vi "TestObserveString_ValueHi.vi"(8 "error in (no error)":errorcluster, 11 "TestCase in":refnum<class "TestObservableData.lvclass">) -> (0 "error out":errorcluster, 3 "TestCase out":refnum<class "TestObservableData.lvclass">)   [LabVIEW 2015, in "TestObservableData.lvclass"]
uses:
  TestObservableData.lvclass
  TestObservableData.lvclass/TestObservableData.ctl
  Framework/IMediator/IMediator Messages/Subscribe Msg/Subscribe Msg.lvclass/Subscribe Msg.ctl
  <vilib>/ActorFramework/Message Enqueuer/Message Enqueuer.lvclass/Message Enqueuer.ctl
  <vilib>/ActorFramework/Message Enqueuer/Enqueue.vi
  <vilib>/ActorFramework/Message Priority Queue/Priority Enqueue.vi
  Framework/IMediator/IMediator Messages/Subscribe Msg/Subscribe Msg.lvclass
  Framework/IMediator/SubscriptionRequest/SubscriptionRequest.lvclass
  Framework/IMediator/ISubscriptionPolicy/ISubscriptionPolicy.lvclass
  Framework/Mediator/Transport/TerminalBinding/TerminalBinding.lvclass
panel:
  out "ControlTerminal":string
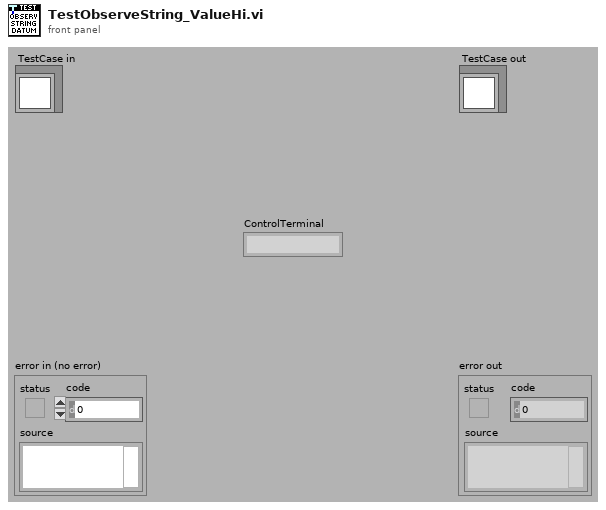
[diagram p1: front panel]
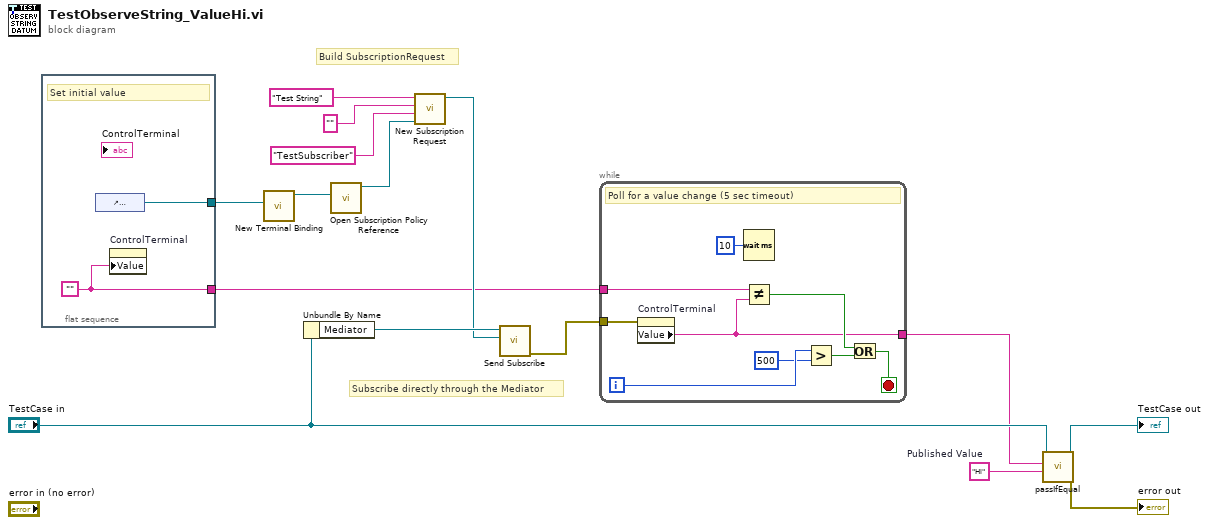
[diagram p0: block diagram]
diagram:
  w1 = "Hi"  # Published Value
  # "Build SubscriptionRequest"
  # "Subscribe directly through the Mediator"
  n1 = flat-sequence {
    tunnel: [w17] -> w5
    tunnel: [w16] -> w3
    frame #0 {
      w16 = "" ("ControlTerminal")
      # "Set initial value"
      n2 = control-ref of="ControlTerminal"() -> (w17:refnum<vi>)
      n3 = property on="ControlTerminal" class="Str"("Value"=w16) -> ()  [unwired: 2 in, 2 out]
    }
  }
  n4 = call "New Terminal Binding.vi"("Ctl Refnum"=w5) -> ("TerminalBinding out"=w6:refnum<class "TerminalBinding.lvclass">)  [unwired: 9 in, 1 out]
  n5 = Unbundle By Name("TestCase in") -> ("Mediator"=w12:refnum<class "Message Enqueuer.lvclass">)
  n6 = call "Open Subscription Policy Reference.vi"("Transport"=w6) -> ("Subscription Policy"=w7:refnum<data-value>)  [unwired: 9 in, 1 out]
  n7 = call "New Subscription Request.vi"("Subscription Policy"=w7, "Unique Subscriber ID"="TestSubscriber", "Type"="", "Topic Name"="Test String") -> ("SubscriptionRequest"=w11:refnum<class "SubscriptionRequest.lvclass">)  [unwired: 7 in]
  n8 = call "Send Subscribe.vi"("Subscription Request"=w11, "Message Enqueuer"=w12) -> ("error out"=w4:errorcluster)  [unwired: 8 in, 1 out]
  n9 = while {
    tunnel: w4 -> [w26]
    tunnel: w3 -> [w25]
    tunnel: [w18] -> w2
    i -> [w21]
    stop <- w19 stop-if-true
    # "Poll for a value change (5 sec timeout)"
    n10 = property on="ControlTerminal" class="Str"(error in=w26) -> ("Value"=w18:string)  [unwired: 1 in, 2 out]
    n11 = Wait (ms)(milliseconds to wait=u32 10) -> ()  [unwired: 1 out]
    n12 = Not Equal?(x=w25, y=w18) -> (x != y?=w24:bool)
    n13 = Greater?(x=w21, y=500) -> (0:w22:bool)
    n14 = Or(x=w24, y=w22) -> (x .or. y?=w19:bool)
  }
  n15 = call-dynamic "passIfEqual.vi"("y"=w1, "x"=w2, "TestCase in"="TestCase in") -> ("error out"=→"error out":errorcluster, "TestCase out"=→"TestCase out":refnum<class "TestObservableData.lvclass">)  [unwired: 7 in]
